vi "Shooter Pusher.vi"(7 "Joystick Trigger":bool=TRUE, 8 "Shoot Pusher Input":enum16{"In", "Extending", "Retracting"}(ring), 9 "Ready?":bool=TRUE, 10 "Extend Time (s)":dbl, 11 "Retract Time (s)":dbl) -> (0 "Shoot Pusher Output":enum16{"In", "Extending", "Retracting"}(ring), 3 "Solenoid Output":T1)   [LabVIEW 2012]
uses:
  <vilib>/Rock Robotics/WPI/Solenoid/WPI_SolenoidValue.ctl
panel:
  out "State":string
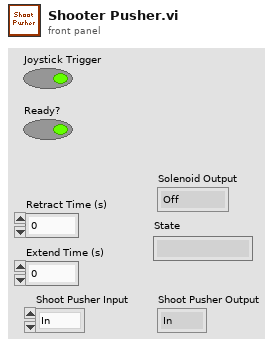
[diagram p1: front panel]
types:
  T1 = typedef "WPI_SolenoidValue.ctl" = enum16{"Off", "On", "Forward", "Reverse"}
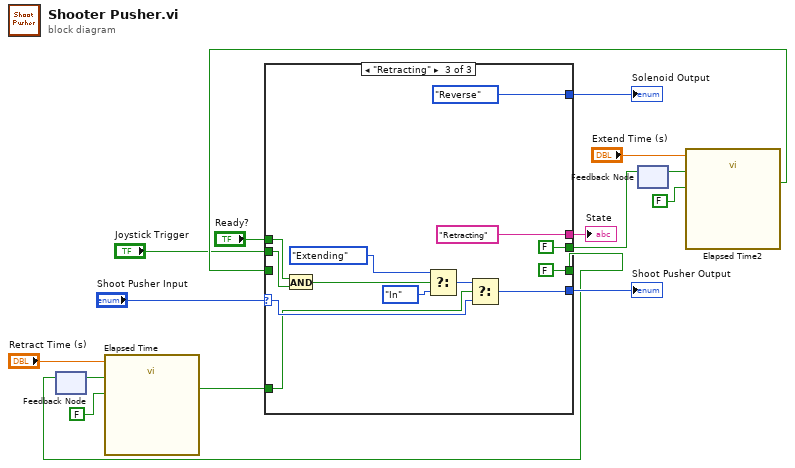
[diagram p0: block diagram]
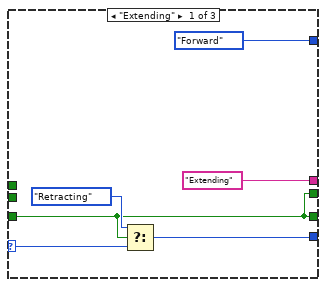
[diagram p2: hidden frame]
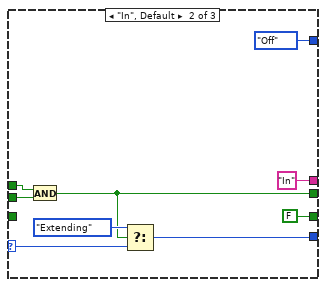
[diagram p3: hidden frame]
diagram:
  n1 = feedback #1() -> (w11:bool)  [unwired: 1 in]
  n2 = call "Elapsed Time"("Time Target (s)"="Retract Time (s)", "Reset"=w11, "Auto Reset"=FALSE) -> ("Time has Elapsed"=w13:bool)  [unwired: 9 in, 7 out]
  n3 = feedback #2() -> (w7:bool)  [unwired: 1 in]
  n4 = call "Elapsed Time2"("Time Target (s)"="Extend Time (s)", "Reset"=w7, "Auto Reset"=FALSE) -> ("Time has Elapsed"=w9:bool)  [unwired: 9 in, 7 out]
  n5 = case shown="\"Retracting\"" "Shoot Pusher Input" {
    selector: "Shoot Pusher Input" -> [w21 w27 w41]
    tunnel: "Joystick Trigger" -> [_ w30 w43]
    tunnel: "Ready?" -> [_ w31 w44]
    tunnel: [w19 w28 w38] -> w16
    tunnel: ["Extending" ("State") "In" ("State") "Retracting" ("State")] -> w15
    tunnel: w13 -> [_ _ w36]
    tunnel: [w18 FALSE FALSE ("Time has Elapsed")] -> w12
    tunnel: w9 -> [w18 _ _]
    tunnel: [w18 w25 FALSE ("Time has Elapsed")] -> w8
    tunnel: [WPI_SolenoidValue."Forward" ("Value") WPI_SolenoidValue."Off" ("Value") WPI_SolenoidValue."Reverse" ("Value")] -> w6
    frame "Extending" {
      n6 = Select(t=enum16{"In", "Extending", "Retracting"}."Retracting", s=w18, f=w21) -> (s? t:f=w19:enum16{"In", "Extending", "Retracting"})
    }
    frame "In", Default {
      n7 = And(x=w31, y=w30) -> (x .and. y?=w25:bool)
      n8 = Select(t=enum16{"In", "Extending", "Retracting"}."Extending", s=w25, f=w27) -> (s? t:f=w28:enum16{"In", "Extending", "Retracting"})
    }
    frame "Retracting" {
      n9 = And(x=w44, y=w43) -> (x .and. y?=w35:bool)
      n10 = Select(t=enum16{"In", "Extending", "Retracting"}."Extending", s=w35, f=enum16{"In", "Extending", "Retracting"}."In") -> (s? t:f=w39:enum16{"In", "Extending", "Retracting"})
      n11 = Select(t=w39, s=w36, f=w41) -> (s? t:f=w38:enum16{"In", "Extending", "Retracting"})
    }
  }
  "State" <- w15
  "Shoot Pusher Output" <- w16
  "Solenoid Output" <- w6
  n12 = feedback-in #1(w12) -> ()
  n13 = feedback-in #2(w8) -> ()
